vi "Bring Timelapse window to front.vi"() -> ()   [LabVIEW 2013]
uses:
  Globals/gl_Time series viewer globals.vi
panel:
  in  "milliseconds to wait":u32=150
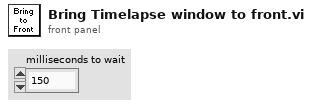
[diagram p1: front panel]
types:
  T1 = typedef "Timelapse viewer refs.ctl" = cluster{"This VI":refnum<vi>, "AVI Mode ind":refnum<vi>, "Play":refnum<vi>, "Stop":refnum<vi>, "Back":refnum<vi>, "Scrollbar":refnum<vi>, "Video length info":refnum<vi>, "Expected speed values":refnum<vi>, "Intensity":refnum<vi>, "Path":refnum<vi>, "Selection sliders":refnum<vi>, "Speed Graph ref":refnum<vi>, "Frame rate set (fps)":refnum<vi>}
  T2 = enum32{"Invalid", "Standard", "Closed", "Hidden", "Minimized", "Maximized"}
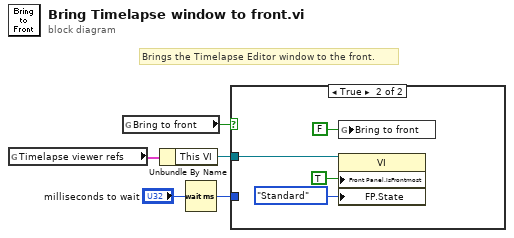
[diagram p0: block diagram]
diagram:
  # "Brings the Timelapse Editor window to the front."
  n1 = global read "gl_Time series viewer globals.vi" "Timelapse viewer refs"() -> (w4:T1)
  n2 = global read "gl_Time series viewer globals.vi" "Bring to front"() -> (w3:bool)
  n3 = Unbundle By Name(w4) -> ("This VI"=w5:refnum<vi>)
  n4 = Wait (ms)(milliseconds to wait="milliseconds to wait") -> (millisecond timer value=w2:u32)
  n5 = case shown="True" w3 {
    tunnel: w5 -> [_ w7]
    tunnel: w2 -> [_ _]
    frame False {
    }
    frame True {
      n6 = global write "gl_Time series viewer globals.vi" "Bring to front"(FALSE ("Bring Timelapse Editor to front")) -> ()
      n7 = property class="VI"(reference=w7, "Front Panel.IsFrontmost"=TRUE ("Front Panel Window:Is Frontmost"), "FP.State"=T2."Standard" ("Front Panel Window:State")) -> ()  [unwired: 1 in, 2 out]
    }
  }
